vi "Server.vi"() -> ()   [LabVIEW 2015]
uses:
  <vilib>/Instr/_visa.llb/VISA Configure Serial Port (Instr).vi
panel:
  out "VISA":string
  out "Remote Information":string
  out "Information":string
  in  "baud rate (9600)":u32=115200
  out "IP Address of remote PC":string
  out "Error out":errorcluster
  out "Remote Command":string
  out "IIP Address of this PC":string
  out "Domain":string
  out "remote port":u16
  out "Domain of remote PC":string
  in  "Port for connection":u16=22022
  in  "Stop SIm":bool
  out "Error out VISA":errorcluster
  out "Feedback":string
  out "Board on port":refnum<visa-resource-name>
  out "Board Status":bool
  in  "instr name":string="Arduino" caption="Board Name"
  # "Server"
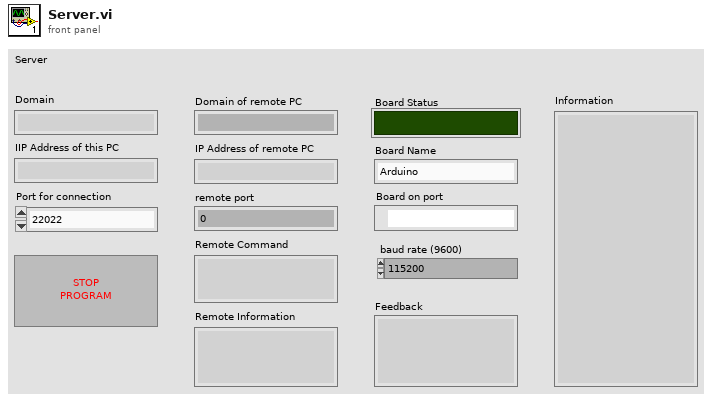
[diagram p1: front panel]
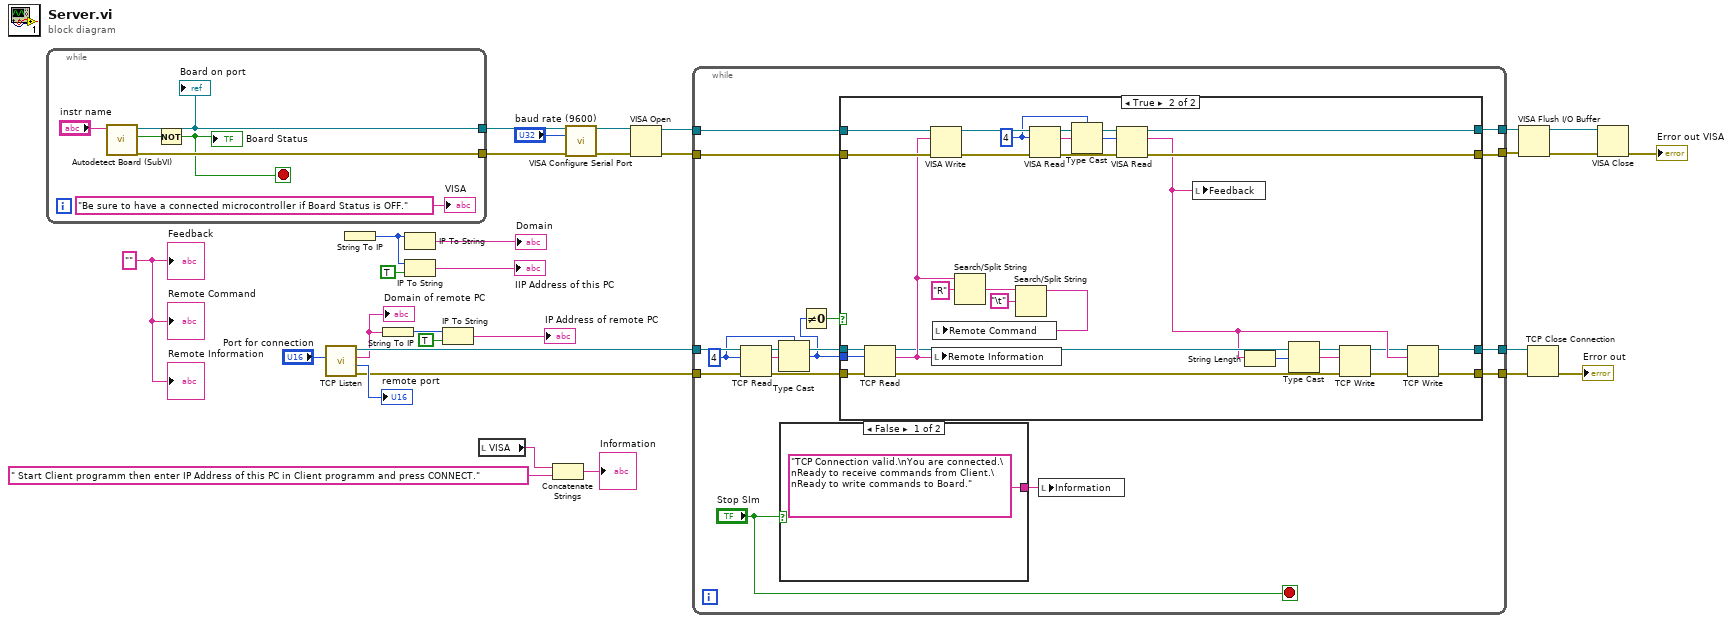
[diagram p0: block diagram]
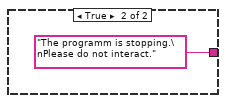
[diagram p3: hidden frame]
diagram:
  w4 = ""
  n1 = while {
    tunnel: [w35] -> w15
    tunnel: [w34] -> w14
    stop <- w33 stop-if-true
    n2 = call "Autodetect Board (SubVI).vi"("instr name"="instr name") -> ("error out"=w34:errorcluster, "status"=w36:bool, "VISA Refnum out"=w35:refnum<visa-resource-name>)  [unwired: 8 in]
    "Board on port" <- w35
    n3 = Not(x=w36) -> (.not. x?=w33:bool)
    "Board Status" <- w33
    "VISA" <- "Be sure to have a connected microcontroller if Board Status is OFF."
  }
  n4 = call <vilib>:"TCP Listen.vi"("port"="Port for connection") -> ("error out"=w22:errorcluster, "remote port"=→"remote port":u16, "remote address"=w19:string, "connection ID"=w23:refnum<k5>)  [unwired: 6 in, 1 out]
  "Domain of remote PC" <- w19
  n5 = String To IP() -> (0:w27:u32)  [unwired: 1 in]
  n6 = String To IP(1:w19) -> (0:w17:u32)
  n7 = IP To String(2:w27) -> (0:→"Domain":string)  [unwired: 1 in]
  n8 = IP To String(1:TRUE ("dot notation? (F)"), 2:w27) -> (0:→"IIP Address of this PC":string)
  n9 = IP To String(1:TRUE ("dot notation? (F)"), 2:w17) -> (0:→"IP Address of remote PC":string)
  n10 = local read "VISA"() -> (w2:string)
  n11 = Concatenate Strings(w2, " Start Client programm then enter IP Address of this PC in Client programm and press CONNECT.") -> (→"Information":string)
  n12 = call-poly "VISA Configure Serial Port"("VISA resource name"=w15, "baud rate (9600)"="baud rate (9600)", "error in (no error)"=w14) -> ("VISA resource name out"=w8:refnum<visa-resource-name>, "error out"=w7:errorcluster)  [unwired: 11 in]
  n13 = VISA Open(error in (no error)=w7, VISA resource name=w8) -> (VISA resource name=w31:refnum<visa-resource-name>, error out=w30:errorcluster)  [unwired: 3 in]
  n14 = while {
    tunnel: w31 -> [w53]
    tunnel: [w41] -> w12
    tunnel: w30 -> [w52]
    tunnel: [w40] -> w11
    tunnel: w23 -> [w51]
    tunnel: [w49] -> w21
    tunnel: w22 -> [w50]
    tunnel: [w48] -> w20
    stop <- "Stop SIm" stop-if-true
    w43 = 4
    n15 = TCP Read(connection ID=w51, bytes to read=w43, error in (no error)=w50) -> (connection ID out=w46:refnum<k5>, data out=w44:string, error out=w45:errorcluster)  [unwired: 2 in]
    n16 = Type Cast(type=w43, x=w44) -> (*(type *) &x=w38:i32)
    n17 = case shown="False" "Stop SIm" {
      tunnel: ["TCP Connection valid.\nYou are connected.\nReady to receive commands from Client.\nReady to write commands to Board." "The programm is stopping.\nPlease do not interact."] -> w47
      frame False {
      }
      frame True {
      }
    }
    n18 = Not Equal To 0?(x=w38) -> (x != 0?=w39:bool)
    n19 = case shown="True" w39 {
      tunnel: w53 -> [w57 w85]
      tunnel: w52 -> [w56 w84]
      tunnel: [w55 w64] -> w49
      tunnel: [w54 w63] -> w48
      tunnel: w46 -> [w55 w80]
      tunnel: w45 -> [w54 w79]
      tunnel: w38 -> [_ w78]
      tunnel: [w57 w66] -> w41
      tunnel: [w56 w65] -> w40
      frame False {
      }
      frame True {
        w72 = 4
        n20 = TCP Read(connection ID=w80, bytes to read=w78, error in (no error)=w79) -> (connection ID out=w71:refnum<k5>, data out=w76:string, error out=w70:errorcluster)  [unwired: 2 in]
        n21 = VISA Write(VISA resource name=w85, write buffer=w76, error in (no error)=w84) -> (VISA resource name out=w75:refnum<visa-resource-name>, error out=w74:errorcluster)  [unwired: 1 out]
        n22 = local write "Remote Information"(w76) -> ()
        n23 = Search/Split String(string=w76, search string/char (-)="R") -> (match + rest of string=w81:string)  [unwired: 1 in, 2 out]
        n24 = Search/Split String(string=w81, search string/char (-)="\t") -> (substring before match=w77:string)  [unwired: 1 in, 2 out]
        n25 = local write "Remote Command"(w77) -> ()
        n26 = VISA Read(VISA resource name=w75, byte count=w72, error in (no error)=w74) -> (VISA resource name out=w69:refnum<visa-resource-name>, read buffer=w73:string, error out=w68:errorcluster)  [unwired: 1 out]
        n27 = Type Cast(type=w72, x=w73) -> (*(type *) &x=w67:i32)
        n28 = VISA Read(VISA resource name=w69, byte count=w67, error in (no error)=w68) -> (VISA resource name out=w66:refnum<visa-resource-name>, read buffer=w62:string, error out=w65:errorcluster)  [unwired: 1 out]
        n29 = local write "Feedback"(w62) -> ()
        n30 = String Length(string=w62) -> (length=w58:i32)
        n31 = Type Cast(x=w58) -> (*(type *) &x=w61:string)  [unwired: 1 in]
        n32 = TCP Write(connection ID=w71, data in=w61, error in (no error)=w70) -> (connection ID out=w60:refnum<k5>, error out=w59:errorcluster)  [unwired: 1 in, 1 out]
        n33 = TCP Write(connection ID=w60, data in=w62, error in (no error)=w59) -> (connection ID out=w64:refnum<k5>, error out=w63:errorcluster)  [unwired: 1 in, 1 out]
      }
    }
    n34 = local write "Information"(w47) -> ()
  }
  n35 = VISA Flush I/O Buffer(VISA resource name=w12, error in (no error)=w11) -> (VISA resource name out=w10:refnum<visa-resource-name>, error out=w9:errorcluster)  [unwired: 1 in]
  n36 = TCP Close Connection(connection ID=w21, error in (no error)=w20) -> (error out=→"Error out":errorcluster)  [unwired: 1 in, 1 out]
  n37 = VISA Close(VISA resource name=w10, error in (no error)=w9) -> (error out=→"Error out VISA":errorcluster)
  "Feedback" <- w4
  "Remote Command" <- w4
  "Remote Information" <- w4
